vi "Typecast Refnum to Queue.vi"(11 "refnum in":refnum<k1>) -> (3 "queue out":refnum<queue>)   [LabVIEW 2017, in "NI_LVConfig.lvlib"]
uses:
  NI_LVConfig.lvlib
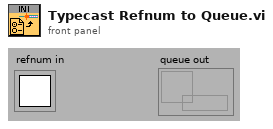
[diagram p1: front panel]
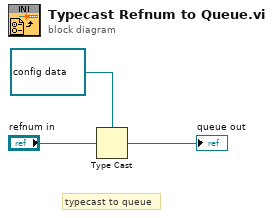
[diagram p0: block diagram]
diagram:
  # "typecast to queue"
  n1 = Type Cast(type=refnum<queue> refnum ("queue out"), x="refnum in") -> (*(type *) &x=→"queue out":refnum<queue>)
